vi "TakeSubstringFromStart.vi"(2 "offset":i32, 3 "string":string) -> (0 "string before offset":string, 1 "string after offset":string)   [LabVIEW 2009]
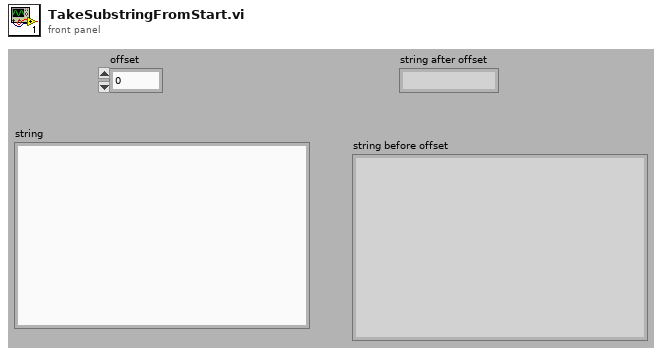
[diagram p1: front panel]
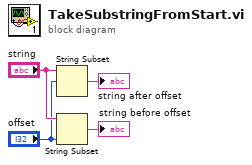
[diagram p0: block diagram]
diagram:
  n1 = String Subset(string="string", offset (0)="offset") -> (substring=→"string after offset":string)  [unwired: 1 in]
  n2 = String Subset(string="string", length (rest)="offset") -> (substring=→"string before offset":string)  [unwired: 1 in]
